vi "Update List.vi"(0 "ListBox":refnum<vi>, 7 "State":T1={"Prompt"="Click to add", "Listbox"=refnum, "Required"={"Strings"=[], "Bottom"=FALSE, "Italic"=FALSE, "FG"=0, "BG"=16777215, "Bold"=FALSE}, "Items"=[], "Req'd"=[], "Events"={"Items Changed"=refnum, "List Changed"=refnum}, "Max Rows"=-1, "Default name"=""}, 11 "Row":i32) -> (4 "reference out":refnum<vi>)   [LabVIEW 2020, in "KListboxEx.xctl"]
uses:
  KListboxEx.xctl
  State.ctl
  Required.ctl
  Events.ctl
  Event Action.ctl
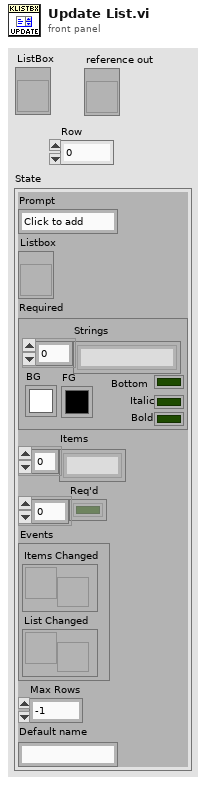
[diagram p1: front panel]
types:
  T1 = typedef "KListboxEx.xctl/State.ctl" = cluster{"Prompt":string, "Listbox":refnum<vi>, "Required":T2, "Items":string[], "Req'd":bool[], "Events":T3, "Max Rows":i32, "Default name":string}
  T2 = typedef "KListboxEx.xctl/Required.ctl" = cluster{"Strings":string[], "Bottom":bool, "Italic":bool, "FG":u32, "BG":u32, "Bold":bool}
  T3 = typedef "KListboxEx.xctl/Events.ctl" = cluster{"Items Changed":refnum<user-event>, "List Changed":refnum<user-event>}
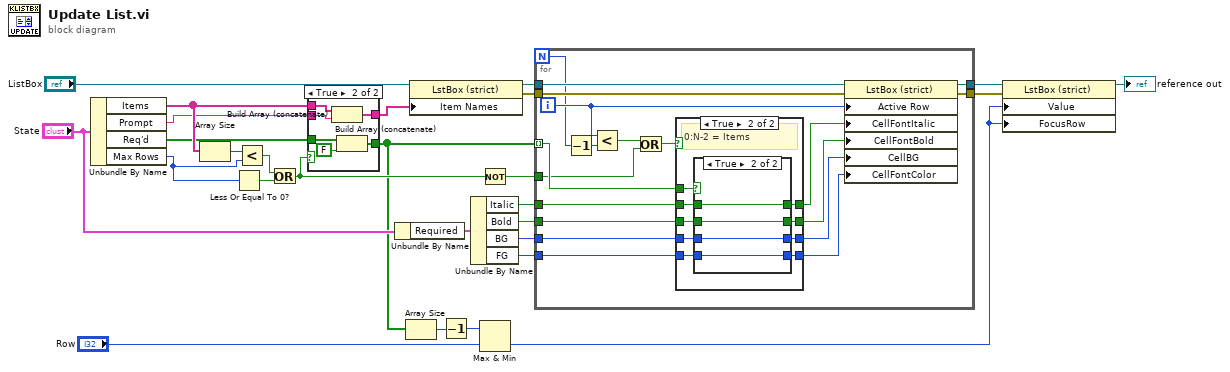
[diagram p0: block diagram]
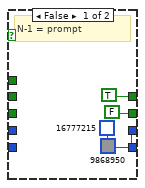
[diagram p3: hidden frame]
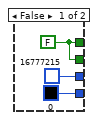
[diagram p4: hidden frame]
diagram:
  n1 = Unbundle By Name("State") -> ("Items"=w9:string[], "Prompt"=w7:string, "Req'd"=w6:bool[], "Max Rows"=w13:i32)
  n2 = Array Size(array=w9) -> (size(s)=w14:i32)
  n3 = Less Or Equal To 0?(x=w13) -> (x <= 0?=w11:bool)
  n4 = Less?(x=w14, y=w13) -> (x < y?=w12:bool)
  n5 = Or(x=w12, y=w11) -> (x .or. y?=w8:bool)
  n6 = case shown="True" w8 {
    tunnel: w9 -> [w29 w35]
    tunnel: [w29 w34] -> w10
    tunnel: w7 -> [_ w33]
    tunnel: [w28 w31] -> w2
    tunnel: w6 -> [w28 w30]
    frame False {
    }
    frame True {
      n7 = Build Array (concatenate)(w35, w33) -> (w34:string[])
      n8 = Build Array (concatenate)(w30, FALSE) -> (w31:bool[])
    }
  }
  n9 = Unbundle By Name("State") -> ("Required"=w16:T2)
  n10 = Array Size(array=w2) -> (size(s)=w3:i32)
  n11 = property on="Property Node" class="LstBox (strict)"(reference="ListBox", "Item Names"=w10) -> (reference out=w27:refnum<vi>, error out=w26:errorcluster)  [unwired: 1 in]
  n12 = Decrement(x=w3) -> (x-1=w1:i32)
  n13 = Unbundle By Name(w16) -> ("Italic"=w21:bool, "Bold"=w20:bool, "BG"=w19:u32, "FG"=w18:u32)
  n14 = Not(x=w8) -> (.not. x?=w5:bool)
  n15 = Max & Min(x=w1, y="Row") -> (min(x,y)=w4:i32)  [unwired: 1 out]
  n16 = for {
    N -> [w49]
    tunnel: w27 -> [w54]
    tunnel: w26 -> [w53]
    tunnel: [w48] -> w25
    tunnel: [w47] -> w24
    tunnel: w2 -> [w46] mode=indexing
    tunnel: w21 -> [w45]
    tunnel: w20 -> [w44]
    tunnel: w19 -> [w43]
    tunnel: w18 -> [w42]
    tunnel: w5 -> [w36]
    i -> [w51]
    n17 = Decrement(x=w49) -> (x-1=w50:i32)
    n18 = Less?(x=w51, y=w50) -> (x < y?=w52:bool)
    n19 = Or(x=w52, y=w36) -> (x .or. y?=w37:bool)
    n20 = case shown="True" w37 {
      tunnel: w46 -> [_ w67]
      tunnel: w45 -> [_ w66]
      tunnel: w44 -> [_ w65]
      tunnel: w43 -> [_ w64]
      tunnel: w42 -> [_ w63]
      tunnel: [TRUE w62] -> w41
      tunnel: [FALSE ("Bold") w61] -> w40
      tunnel: [u32 16777215 w60] -> w39
      tunnel: [u32 9868950 w59] -> w38
      frame False {
        # "N-1 = prompt"
      }
      frame True {
        # "0:N-2 = Items"
        n21 = case shown="True" w67 {
          tunnel: w66 -> [_ w74]
          tunnel: w65 -> [_ w73]
          tunnel: w64 -> [_ w72]
          tunnel: w63 -> [_ w71]
          tunnel: [w70 w74] -> w62
          tunnel: [w70 w73] -> w61
          tunnel: [u32 16777215 w72] -> w60
          tunnel: [u32 0 w71] -> w59
          frame False {
            w70 = FALSE ("Italic")
          }
          frame True {
          }
        }
      }
    }
    n22 = property on="Property Node" class="LstBox (strict)"(reference=w54, error in=w53, "Active Row"=w51, "CellFontItalic"=w41, "CellFontBold"=w40, "CellBG"=w39, "CellFontColor"=w38) -> (reference out=w48:refnum<vi>, error out=w47:errorcluster)
  }
  n23 = property on="Property Node" class="LstBox (strict)"(reference=w25, error in=w24, "Value"=w4, "FocusRow"=w4) -> (reference out=→"reference out":refnum<vi>)  [unwired: 1 out]
